vi "CleanUp Diagram.vi"(8 "error in (no error)":errorcluster, 10 "Top Level Diagram":refnum<vi>, 11 "Structures in":refnum<class "Structures.lvclass">) -> (0 "error out":errorcluster, 3 "Structures out":refnum<class "Structures.lvclass">)   [LabVIEW 2025, in "Structures.lvclass"]
doc: "Find all the main objects and run block diagram cleanup on that main object."
uses:
  Structures.lvclass
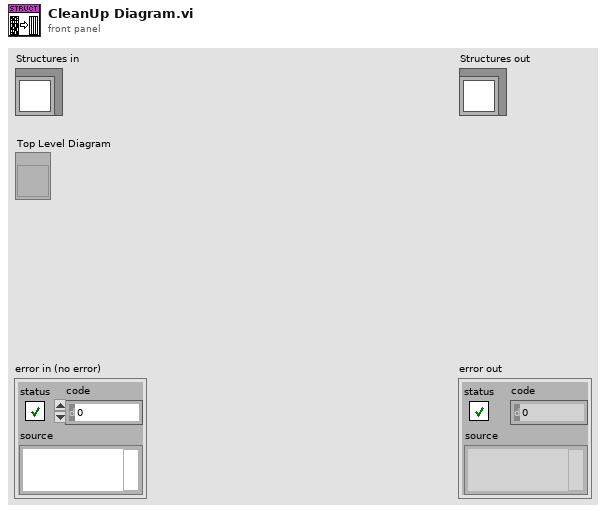
[diagram p1: front panel]
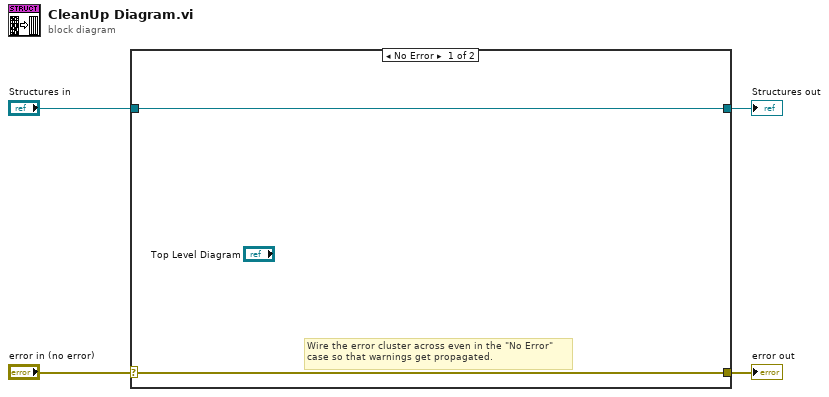
[diagram p0: block diagram]
diagram:
  n1 = case shown="No Error" "error in (no error)" {
    selector: "error in (no error)" -> [w5 w8]
    tunnel: [w5 w8] -> w3
    tunnel: [w6 w7] -> w1
    tunnel: "Structures in" -> [w6 w7]
    frame No Error {
      # "Wire the error cluster across even in the \"No Error\"\ncase so that warnings get propagated."
    }
    frame Error {
    }
  }
  "error out" <- w3
  "Structures out" <- w1
